vi "Read System Status.vi"(8 "error in (no error)":errorcluster, 11 "System Actor in":refnum<class "System Actor.lvclass">) -> (0 "error out":errorcluster, 2 "System Status":T1, 3 "System Actor out":refnum<class "System Actor.lvclass">)   [LabVIEW 2013, in "Robot Actors.lvlib" / "System Actor.lvlib" / "System Actor.lvclass"]
uses:
  System Actor.lvclass
  System Status.ctl
  Command/Command Class/Command Status.ctl
  Command/Command Class/Command States.ctl
  System Actor.lvclass/System Actor.ctl
  Command/Command Class/Command.lvclass
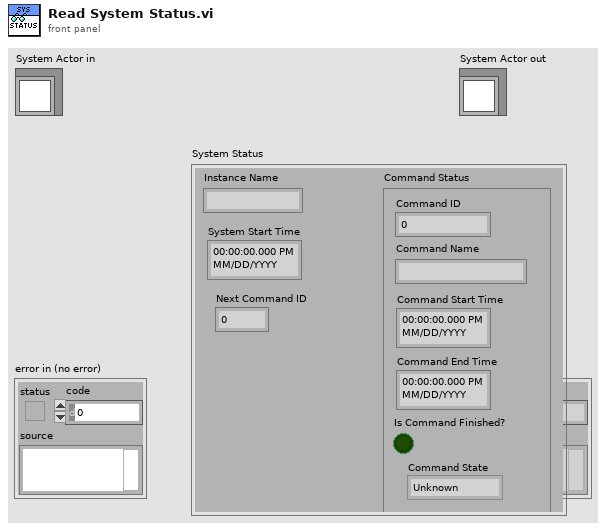
[diagram p1: front panel]
types:
  T1 = typedef "Robot Actors.lvlib/System Actor.lvlib/System Actor.lvclass/System Status.ctl" = cluster{"Instance Name":string, "Command Status":T2, "System Start Time":timestamp, "Next Command ID":dbl}
  T2 = typedef "Robot Actors.lvlib/Command.lvlib/Command.lvclass/Command Status.ctl" = cluster{"Command Name":string, "Command Start Time":timestamp, "Command End Time":timestamp, "Is Command Finished?":bool, "Command ID":dbl, "Command State":T3}
  T3 = typedef "Robot Actors.lvlib/Command.lvlib/Command.lvclass/Command States.ctl" = enum16{"Unknown", "Started", "Stopped", "Finished"}
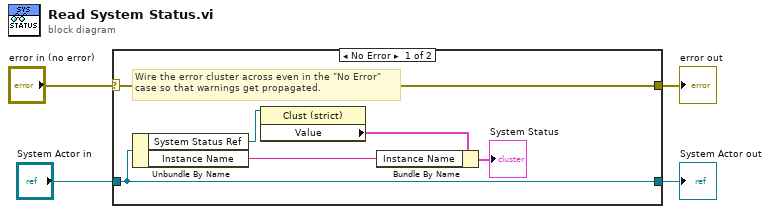
[diagram p0: block diagram]
diagram:
  n1 = case shown="No Error" "error in (no error)" {
    selector: "error in (no error)" -> [w10 w12]
    tunnel: [w10 w12] -> w3
    tunnel: [w9 w11] -> w1
    tunnel: "System Actor in" -> [w9 w11]
    frame No Error {
      # "Wire the error cluster across even in the \"No Error\"\ncase so that warnings get propagated."
      n2 = Unbundle By Name(w9) -> ("System Status Ref"=w8:refnum<vi>, "Instance Name"=w5:string)
      n3 = property class="Clust (strict)"(reference=w8) -> ("Value"=w7:T1)  [unwired: 1 in, 2 out]
      n4 = Bundle By Name(cluster=w7, "Instance Name"=w5) -> (→"System Status":T1)
    }
    frame Error {
    }
  }
  "error out" <- w3
  "System Actor out" <- w1
